vi "Main.vi"() -> ()   [LabVIEW 2016]
uses:
  Tax_calculation.lvclass
  System_Tray_Icon/MenueItem/MenueItem.lvclass
  PublicSubvi/BoolACT.ctl
  System_Tray_Icon/Icon/Icon.lvclass
  System_Tray_Icon/Notifyicon/NotifyIcon.lvclass
  System_Tray_Icon/BallonTip/BalloonTip.lvclass
  System_Tray_Icon/ContexMenue/ContexMenue.lvclass
  Tax_calculation.lvclass/Tax_calculation.ctl
panel:
  out "Menue":string
  out "汇算结果（供参考） 3":string
  out "total_income 2":dbl
  out "汇算结果（供参考） 2":string
  out "total_income":dbl
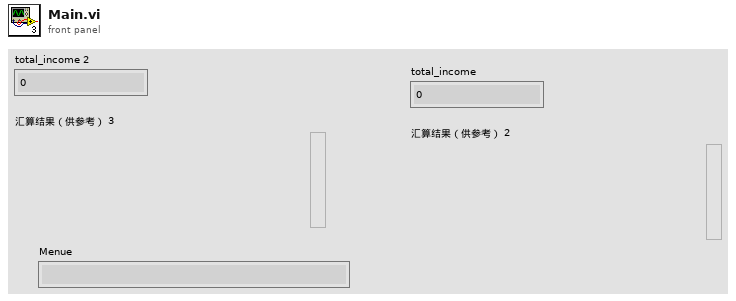
[diagram p1: front panel]
types:
  T1 = typedef "BoolACT.ctl" = enum16{"Get", "Set"}
  T2 = enum32{"Invalid", "Standard", "Closed", "Hidden", "Minimized", "Maximized"}
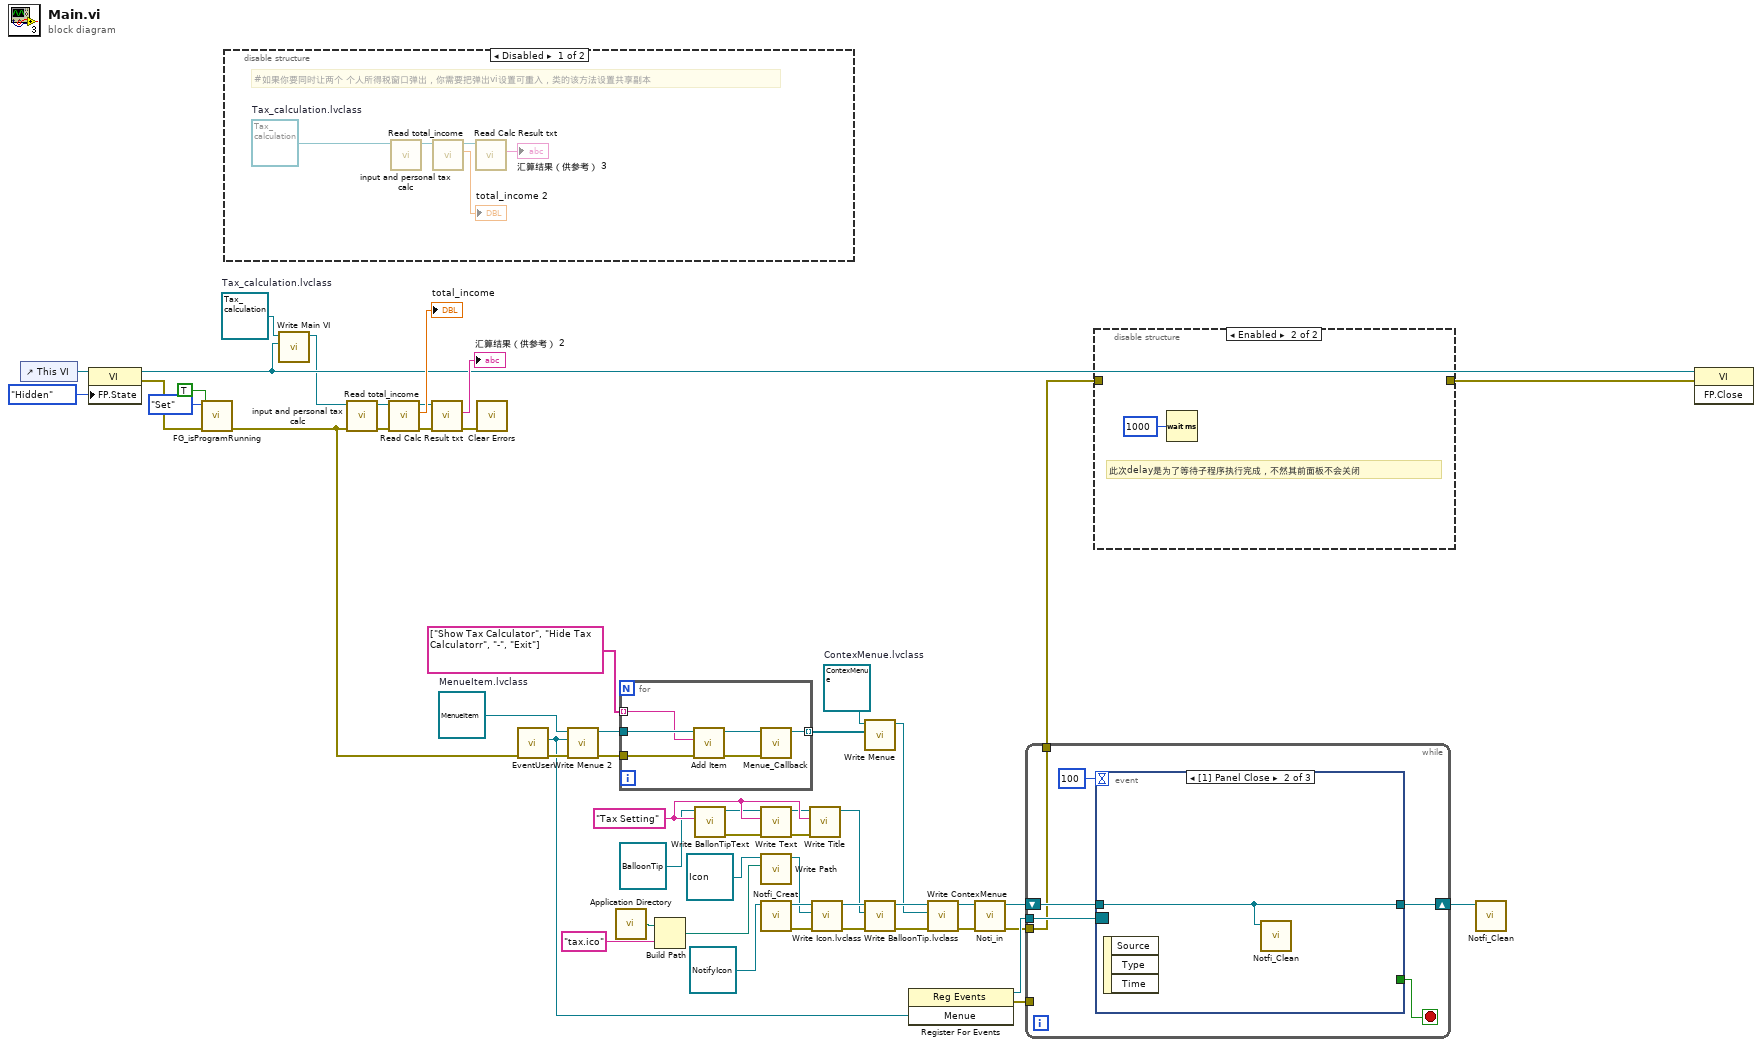
[diagram p0: block diagram]
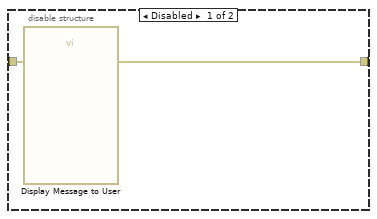
[diagram p2: hidden frame]
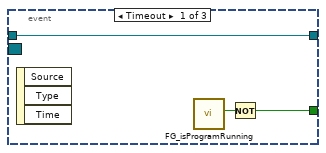
[diagram p3: hidden frame]
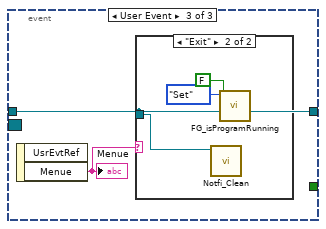
[diagram p4: hidden frame]
diagram:
  w23 = refnum<class "ContexMenue.lvclass"> refnum  # ContexMenue.lvclass
  w29 = "Tax Setting" ("BallonTipText")
  w44 = refnum<class "MenueItem.lvclass"> refnum  # MenueItem.lvclass
  w7 = refnum<class "Tax_calculation.lvclass"> refnum  # Tax_calculation.lvclass
  n1 = control-ref of="This VI"() -> (w49:refnum<vi>)
  n2 = property class="VI"(reference=w49, "FP.State"=T2."Hidden" ("Front Panel Window:State")) -> (reference out=w6:refnum<vi>, error out=w40:errorcluster)  [unwired: 1 in]
  n3 = call "FG_isProgramRunning"("error in (no error)"=w40, "Value"=TRUE, "ACT"=BoolACT."Set") -> ("error out"=w34:errorcluster)  [unwired: 7 in, 1 out]
  n4 = disable-structure shown="Disabled" {
    frame Disabled {
      w54 = refnum<class "Tax_calculation.lvclass"> refnum  # Tax_calculation.lvclass
      # "#如果你要同时让两个 个人所得税窗口弹出，你需要把弹出vi设置可重入，类的该方法设置共享副本"
      n5 = call-dynamic "input and personal tax calc .vi"("Tax_calculation in"=w54) -> ("Tax_calculation out"=w55:refnum<class "Tax_calculation.lvclass">)  [unwired: 9 in, 1 out]
      n6 = call "Read total_income.vi"("Tax_calculation in"=w55) -> ("total_income"=→"total_income 2":dbl, "Tax_calculation out"=w57:refnum<class "Tax_calculation.lvclass">)  [unwired: 8 in, 1 out]
      n7 = call "Read Calc Result txt.vi"("Tax_calculation in"=w57) -> ("汇算结果（供参考）"=→"汇算结果（供参考） 3":string)  [unwired: 8 in, 2 out]
    }
    frame Enabled {
    }
  }
  n8 = call "Write Main VI.vi"("Main VI"=w6, "Tax_calculation in"=w7) -> ("Tax_calculation out"=w5:refnum<class "Tax_calculation.lvclass">)  [unwired: 8 in, 1 out]
  n9 = call-dynamic "input and personal tax calc .vi"("error in (no error)"=w34, "Tax_calculation in"=w5) -> ("error out"=w46:errorcluster, "Tax_calculation out"=w53:refnum<class "Tax_calculation.lvclass">)  [unwired: 8 in]
  n10 = call "Read total_income.vi"("error in (no error)"=w46, "Tax_calculation in"=w53) -> ("error out"=w45:errorcluster, "total_income"=→"total_income":dbl, "Tax_calculation out"=w51:refnum<class "Tax_calculation.lvclass">)  [unwired: 7 in]
  n11 = call "Read Calc Result txt.vi"("error in (no error)"=w45, "Tax_calculation in"=w51) -> ("error out"=w47:errorcluster, "汇算结果（供参考）"=→"汇算结果（供参考） 2":string)  [unwired: 7 in, 1 out]
  n12 = call <vilib>:"Clear Errors.vi"("error in (no error)"=w47) -> ()  [unwired: 5 in, 2 out]
  n13 = call "EventUser.vi"("error in (no error)"=w34) -> ("error out"=w43:errorcluster, "Menue"=w41:refnum<user-event>)  [unwired: 9 in]
  n14 = call-dynamic "Write Menue 2.vi"("error in (no error)"=w43, "Menue 2"=w41, "MenueItem in"=w44) -> ("error out"=w35:errorcluster, "MenueItem out"=w42:refnum<class "MenueItem.lvclass">)  [unwired: 7 in]
  n15 = call <vilib>:"Application Directory.vi"() -> ("Application Directory"=w32:path)
  n16 = for {
    tunnel: w42 -> [w64]
    tunnel: string[] ["Show Tax Calculator", "Hide Tax Calculatorr", "-", "Exit"] ("Array") -> [w62] mode=indexing
    tunnel: w35 -> [w60]
    tunnel: [w59] -> w22 mode=indexing
    n17 = call-dynamic "Add Item.vi"("error in (no error)"=w60, "text"=w62, "MenueItem in"=w64) -> ("error out"=w61:errorcluster, "MenueItem out"=w63:refnum<class "MenueItem.lvclass">)  [unwired: 7 in]
    n18 = call-dynamic "Menue_Callback.vi"("error in (no error)"=w61, "MenueItem in"=w63) -> ("MenueItem out"=w59:refnum<class "MenueItem.lvclass">)  [unwired: 8 in, 1 out]
  }
  n19 = Build Path(base path=w32, name or relative path="tax.ico") -> (appended path=w30:path)
  n20 = call-dynamic "Write BallonTipText.vi"("BallonTipText"=w29, "BalloonTip in"=refnum<class "BalloonTip.lvclass"> refnum ("BalloonTip.lvclass")) -> ("error out"=w28:errorcluster, "BalloonTip out"=w25:refnum<class "BalloonTip.lvclass">)  [unwired: 8 in]
  n21 = call-dynamic "Write Text.vi"("error in (no error)"=w28, "Text"=w29, "BalloonTip in"=w25) -> ("error out"=w27:errorcluster, "BalloonTip out"=w26:refnum<class "BalloonTip.lvclass">)  [unwired: 7 in]
  n22 = call-dynamic "Write Path.vi"("Path"=w30, "Icon in"=refnum<class "Icon.lvclass"> refnum ("Icon.lvclass")) -> ("Icon out"=w14:refnum<class "Icon.lvclass">)  [unwired: 8 in, 1 out]
  n23 = call "Notfi_Creat.vi"("NotifyIcon in"=refnum<class "NotifyIcon.lvclass"> refnum ("NotifyIcon.lvclass")) -> ("error out"=w15:errorcluster, "NotifyIcon out"=w16:refnum<class "NotifyIcon.lvclass">)  [unwired: 9 in]
  n24 = call-dynamic "Write Title.vi"("error in (no error)"=w27, "Title"=w29, "BalloonTip in"=w26) -> ("BalloonTip out"=w13:refnum<class "BalloonTip.lvclass">)  [unwired: 7 in, 1 out]
  n25 = call-dynamic "Write Icon.lvclass.vi"("error in (no error)"=w15, "Icon.lvclass"=w14, "NotifyIcon in"=w16) -> ("error out"=w21:errorcluster, "NotifyIcon out"=w20:refnum<class "NotifyIcon.lvclass">)  [unwired: 7 in]
  n26 = call-dynamic "Write Menue.vi"("Menue"=w22, "ContexMenue in"=w23) -> ("ContexMenue out"=w12:refnum<class "ContexMenue.lvclass">)  [unwired: 8 in, 1 out]
  n27 = call-dynamic "Write BalloonTip.lvclass.vi"("error in (no error)"=w21, "BalloonTip.lvclass"=w13, "NotifyIcon in"=w20) -> ("error out"=w18:errorcluster, "NotifyIcon out"=w19:refnum<class "NotifyIcon.lvclass">)  [unwired: 7 in]
  n28 = register-events(w41) -> (reference out=w36:refnum<event-registration>, error out=w37:errorcluster)  [unwired: 2 in]
  n29 = call-dynamic "Write ContexMenue.vi"("error in (no error)"=w18, "ContexMenue.lvclass"=w12, "NotifyIcon in"=w19) -> ("error out"=w11:errorcluster, "NotifyIcon out"=w10:refnum<class "NotifyIcon.lvclass">)  [unwired: 7 in]
  n30 = call-dynamic "Noti_in.vi"("error in (no error)"=w11, "NotifyIcon in"=w10) -> ("error out"=w8:errorcluster, "NotifyIcon out"=w9:refnum<class "NotifyIcon.lvclass">)  [unwired: 8 in]
  n31 = while {
    tunnel: w37 -> [_]
    tunnel: w36 -> [w68]
    shift-right: [w67] -> w2
    shift-left: w9 -> [w66]
    tunnel: w8 -> [w65]
    tunnel: [w65] -> w4
    stop <- w69 stop-if-true
    n32 = event shown="[1] Panel Close" {
      selector: w68 -> [_ _ _]
      dyn-events: _ -> [_ _ _]
      timeout: 100 -> [_ _ _]
      tunnel: [w72 _ _] -> w69
      tunnel: [w71 w74 w75] -> w67
      tunnel: w66 -> [w71 w74 w75]
      event Timeout {
        n33 = event-data() -> ()  [unwired: 1 in, 3 out]
        n34 = call "FG_isProgramRunning"() -> ("Value"=w73:bool)  [unwired: 10 in, 1 out]
        n35 = Not(x=w73) -> (.not. x?=w72:bool)
      }
      event Panel Close {
        n36 = event-data() -> ()  [unwired: 1 in, 3 out]
        n37 = call-dynamic "Notfi_Clean.vi"("NotifyIcon in"=w74) -> ()  [unwired: 9 in, 2 out]
      }
      event User Event {
        n38 = event-data() -> ("Menue"=w76:string)  [unwired: 1 in, 1 out]
        "Menue" <- w76
        n39 = case shown="\"Exit\"" w76 {
          tunnel: w75 -> [_ w79]
          frame "False", Default {
          }
          frame "Exit" {
            n40 = call-dynamic "Notfi_Clean.vi"("NotifyIcon in"=w79) -> ()  [unwired: 9 in, 2 out]
            n41 = call "FG_isProgramRunning"("Value"=FALSE, "ACT"=BoolACT."Set") -> ()  [unwired: 8 in, 2 out]
          }
        }
      }
    }
  }
  n42 = disable-structure shown="Enabled" {
    disable-tunnel: w4 -> [w81 _]
    disable-tunnel: [w80 _] -> w1
    frame Disabled {
      n43 = call "Display Message to User"("error in (no error)"=w81) -> ("error out"=w80:errorcluster)  [unwired: 9 in, 1 out]
    }
    frame Enabled {
      # "此次delay是为了等待子程序执行完成，不然其前面板不会关闭"
      n44 = Wait (ms)(milliseconds to wait=u32 1000) -> ()  [unwired: 1 out]
    }
  }
  n45 = call-dynamic "Notfi_Clean.vi"("NotifyIcon in"=w2) -> ()  [unwired: 9 in, 2 out]
  n46 = invoke class="VI" method="FP.Close"(reference=w6, error in=w1) -> ()  [unwired: 1 in, 3 out]
